vi "Destroy.vi"(0 "reference":refnum<class "Direction.lvclass">, 5 "error in (no error)":errorcluster) -> (19 "error out":errorcluster)   [LabVIEW 2016, in "Direction.lvclass"]
doc: "Destroys an object created with a Direction constructor VI or a subclass of the Direction class. This VI must be reentrant.\n\n[GOOP 2.1]"
uses:
  <resource>/Framework/Providers/Open_GDS/UML/Direction_class/Direction.lvclass
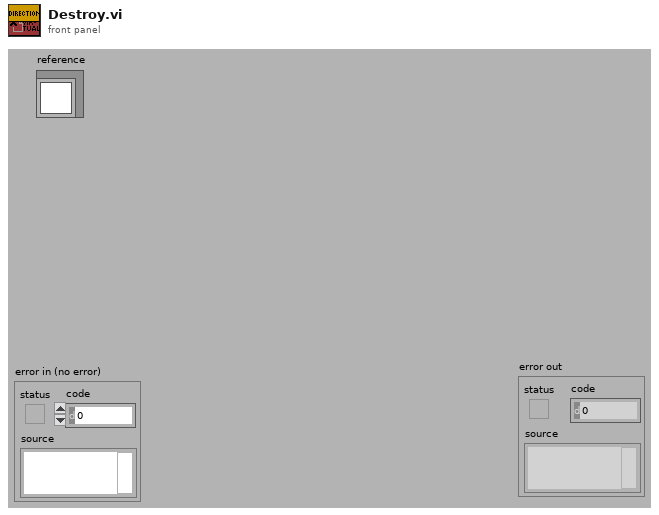
[diagram p1: front panel]
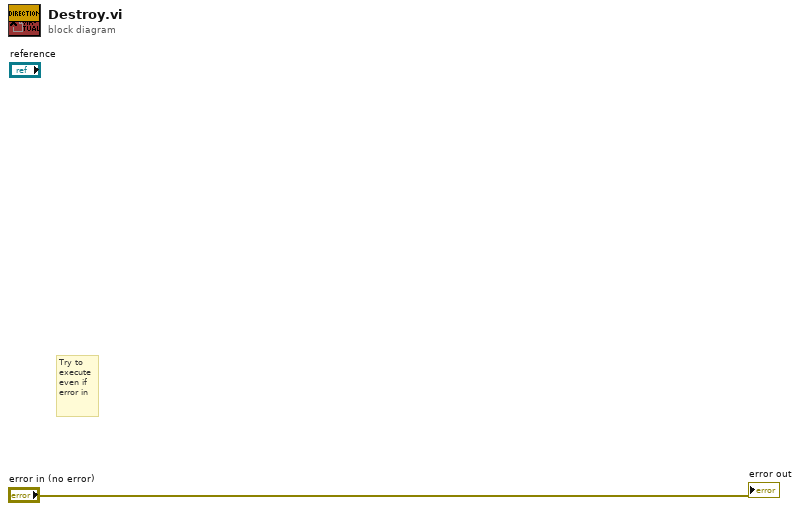
[diagram p0: block diagram]
diagram:
  # "Try to\nexecute\neven if\nerror in"
  "error out" <- "error in (no error)"
